vi "Is Null Token.vi"(1 "Token":T1) -> (0 "Null Token":bool)   [LabVIEW 2020, in "Stream.lvlib" / "URLPattern.lvclass"]
uses:
  URLPattern.lvclass
  Token.ctl
  Token Type.ctl
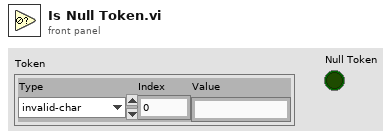
[diagram p1: front panel]
types:
  T1 = typedef "Stream.lvlib/URLPattern.lvclass/Token.ctl" = cluster{"Type":T2, "Index":i32, "Value":string}
  T2 = typedef "Stream.lvlib/URLPattern.lvclass/Token Type.ctl" = enum16{"invalid-char", "open", "close", "regexp", "name", "char", "escaped-char", "other-modifier", "asterisk", "end"}
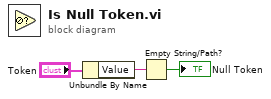
[diagram p0: block diagram]
diagram:
  n1 = Unbundle By Name("Token") -> ("Value"=w2:string)
  n2 = Empty String/Path?(string/path=w2) -> (empty?=→"Null Token":bool)
